vi "Update Inst Config.vi"(8 "error in (no error)":errorcluster, 10 "Data In":string[][](array[string])) -> (0 "error out":errorcluster, 2 "Inst Config Setting":T1={"Current Limit Setting"={"Address"=0.0, "Current Limit"=0.0}, "Over Voltage Setting"={"Address"=0.0, "Over Voltage Limit"=0.0, "Protection Delay"=0.1}, "Connection"={"Ref"=variant, "Parameter"={"Baud Rate"=9600}}} {"Connection"."Parameter"."Baud Rate" items=["300"=300, "600"=600, "1200"=1200, "2400"=2400, "4800"=4800, "9600"=9600, "19200"=19200]; "Over Voltage Setting"."Protection Delay" min=0.1 max=0.6; "Over Voltage Setting"."Over Voltage Limit" min=1.0 max=160.0})   [LabVIEW 2021, in "DC PWS.lvlib"]
uses:
  DC PWS.lvlib
  Inst Config Setting.ctl
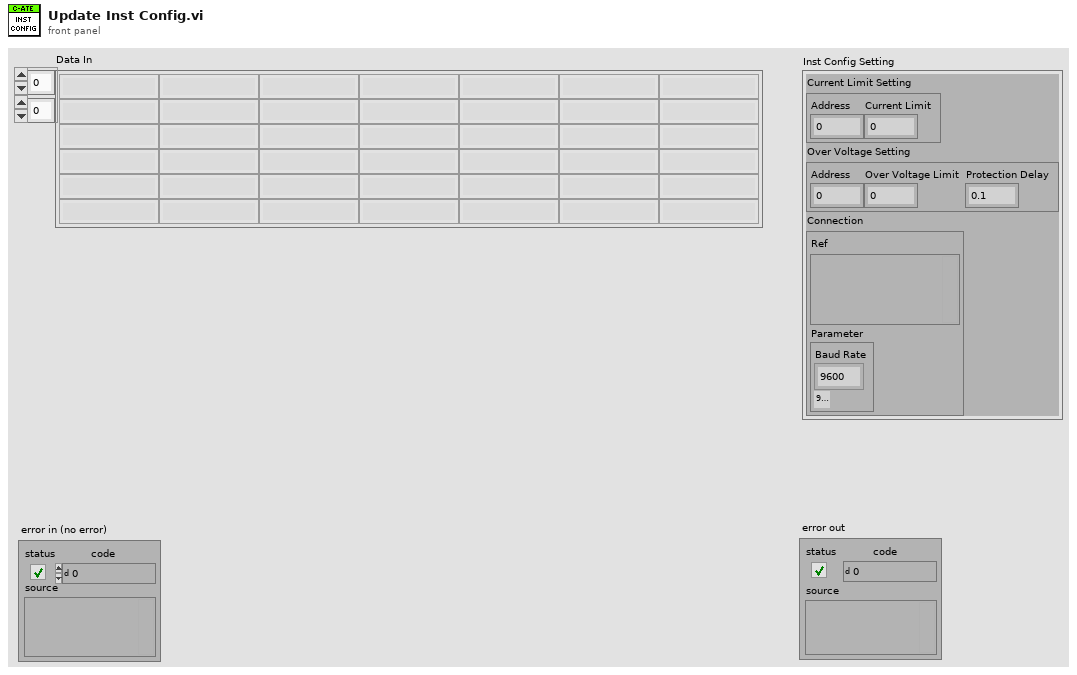
[diagram p1: front panel]
types:
  T1 = typedef "DC PWS.lvlib/Inst Config Setting.ctl" = cluster{"Current Limit Setting":cluster{"Address":dbl, "Current Limit":dbl}, "Over Voltage Setting":cluster{"Address":dbl, "Over Voltage Limit":dbl, "Protection Delay":dbl}, "Connection":cluster{"Ref":variant, "Parameter":cluster{"Baud Rate":u32}}}
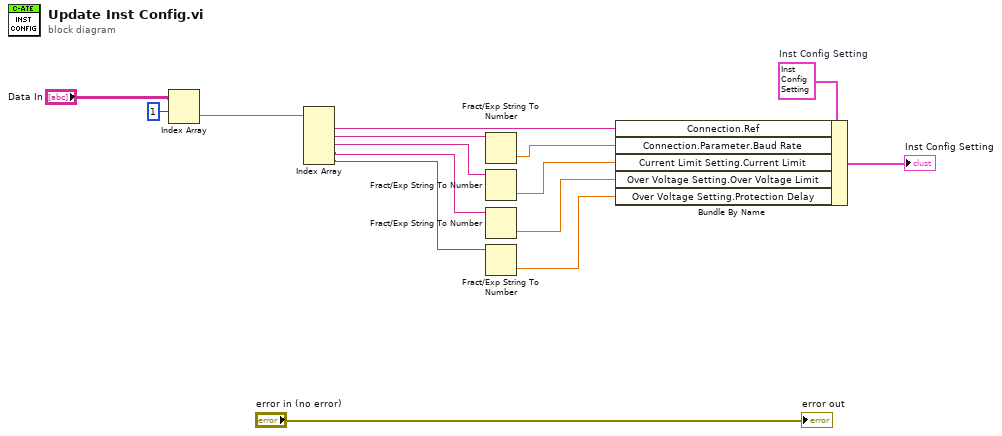
[diagram p0: block diagram]
diagram:
  w12 = T1 {"Current Limit Setting"={"Address"=0.0, "Current Limit"=0.0}, "Over Voltage Setting"={"Address"=0.0, "Over Voltage Limit"=0.0, "Protection Delay"=0.1}, "Connection"={"Ref"=variant(u32 9600), "Parameter"={"Baud Rate"=9600}}}  # Inst Config Setting
  n1 = Index Array(array="Data In", index (row)=1) -> (element=w11:string[])  [unwired: 1 in]
  n2 = Index Array(array=w11) -> (element #1=w10:string, element #2=w9:string, element #3=w7:string, element #4=w5:string, element #5=w4:string)  [unwired: 5 in]
  n3 = Fract/Exp String To Number(string=w9) -> (number=w8:dbl)  [unwired: 3 in, 1 out]
  n4 = Fract/Exp String To Number(string=w7) -> (number=w6:dbl)  [unwired: 3 in, 1 out]
  n5 = Fract/Exp String To Number(string=w5) -> (number=w3:dbl)  [unwired: 3 in, 1 out]
  n6 = Fract/Exp String To Number(string=w4) -> (number=w2:dbl)  [unwired: 3 in, 1 out]
  n7 = Bundle By Name(cluster=w12, "Connection.Ref"=w10, "Connection.Parameter.Baud Rate"=w8, "Current Limit Setting.Current Limit"=w6, "Over Voltage Setting.Over Voltage Limit"=w3, "Over Voltage Setting.Protection Delay"=w2) -> (→"Inst Config Setting":T1)
  "error out" <- "error in (no error)"
